vi "Update User Details.vi"(8 "error in (no error)":errorcluster, 10 "Update Credential":T1, 11 "MySQL in":refnum<class "MySQL.lvclass">) -> (0 "error out":errorcluster, 3 "MySQL out":refnum<class "MySQL.lvclass">)   [LabVIEW 2016, in "Database.lvlib" / "MySQL.lvclass"]
uses:
  MySQL.lvclass
  DB/Update Credential.ctl
  DB/DB.lvclass
  Database.lvlib
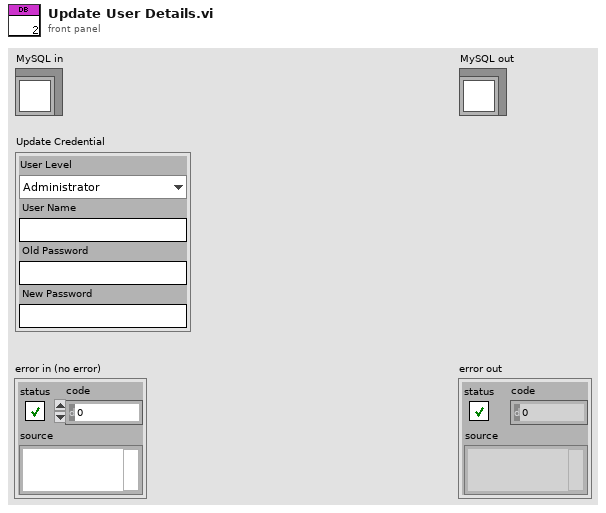
[diagram p1: front panel]
types:
  T1 = typedef "Database.lvlib/Update Credential.ctl" = cluster{"User Level":enum16{"Administrator", "Engineer", "Operator"}, "User Name":string, "Old Password":string, "New Password":string}
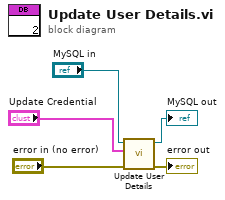
[diagram p0: block diagram]
diagram:
  n1 = call-parent "Update User Details.vi"("error in (no error)"="error in (no error)", "Update Credential"="Update Credential", "DB in"="MySQL in") -> ("error out"=→"error out":errorcluster, "DB out"=→"MySQL out":refnum<class "MySQL.lvclass">)  [unwired: 7 in]
